vi "ReadCSV.vi"(8 "error in (no error)":errorcluster, 11 "file path":path) -> (0 "error out":errorcluster, 3 "Data":string[][](table))   [LabVIEW 2019, in "flashcards.lvlib"]
uses:
  flashcards.lvlib
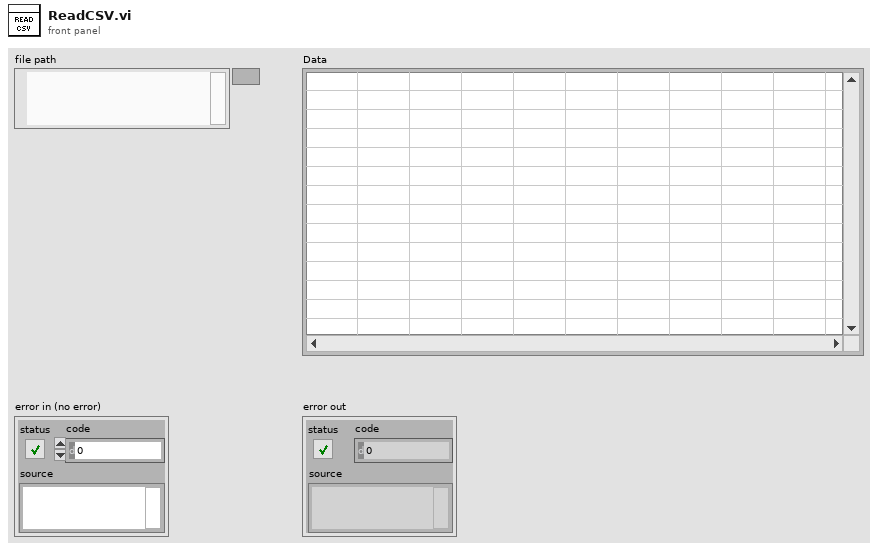
[diagram p1: front panel]
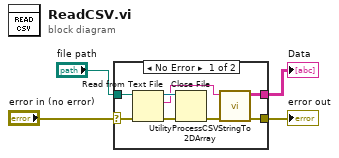
[diagram p0: block diagram]
diagram:
  n1 = case shown="No Error" "error in (no error)" {
    selector: "error in (no error)" -> [w8 w13]
    tunnel: [w7 w13] -> w3
    tunnel: [w6 _] -> w2
    tunnel: "file path" -> [w5 _]
    frame No Error {
      n2 = Read from Text File(file (use dialog)=w5, error in=w8) -> (refnum out=w11:refnum<file>, text=w9:string, error out=w12:errorcluster)  [unwired: 2 in, 1 out]
      n3 = Close File(refnum=w11, error in=w12) -> (error out=w10:errorcluster)  [unwired: 1 out]
      n4 = call "UtilityProcessCSVStringTo2DArray.vi"("error in (no error)"=w10, "CSV String"=w9) -> ("error out"=w7:errorcluster, "Array"=w6:string[][])  [unwired: 8 in]
    }
    frame Error {
    }
  }
  "Data" <- w2
  "error out" <- w3
